vi "case_torture.vi"(7 "Main VI reference":refnum<vi>, 8 "error in (no error)":errorcluster, 10 "queue in":refnum<queue>, 11 "VISA resource name in":refnum<visa-resource-name>) -> (0 "error out":errorcluster, 3 "VISA Refnum out":refnum<visa-resource-name>)   [LabVIEW 2020]
uses:
  controls/message cluster.ctl
  <instrlib>/Marlin Instrument Driver/Public/controls/move parameters.ctl
  6b4587bc-0fd2-4684-895c-966bfeff11c4.vi
  3dbca1fd-0638-40ad-b8cf-a0dccebfc0b9.vi
  16951a91-4322-4001-be28-78344395b4b7.vi
  74ea327f-2ce8-422c-9958-5bfd1753f00f.vi
  50b149f9-9e82-4165-acdf-462a277af1c9.vi
  374137ba-4f25-4847-9236-12953adebbe7.vi
  f821f635-f9e4-4ceb-808f-b90ab8643010.vi
  <instrlib>/Marlin Instrument Driver/Marlin Instrument Driver.lvlib
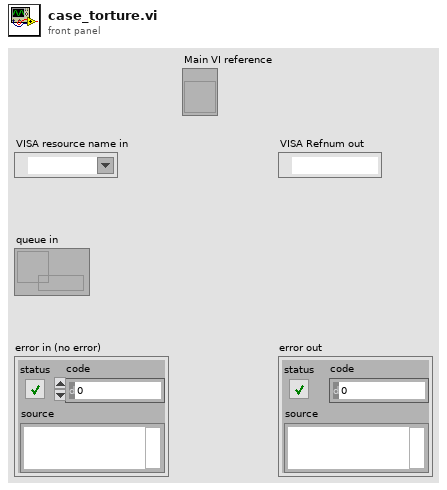
[diagram p1: front panel]
types:
  T1 = typedef "message cluster.ctl" = cluster{"message":string, "data":variant}
  T2 = typedef "Marlin Instrument Driver.lvlib/move parameters.ctl" = cluster{"E":dbl, "F":dbl, "X":dbl, "Y":dbl, "Z":dbl}
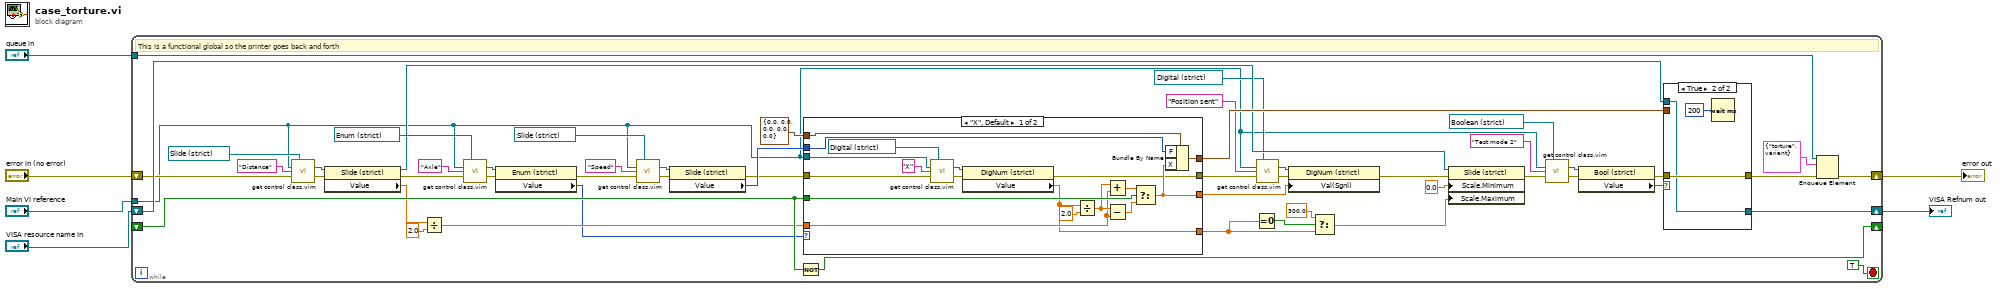
[diagram p0: block diagram]
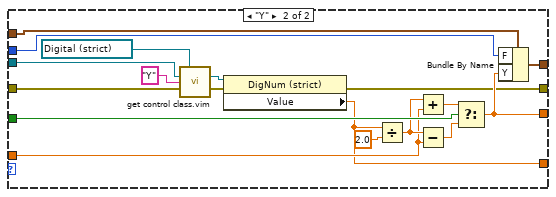
[diagram p2: hidden frame]
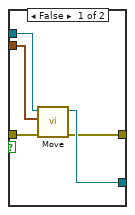
[diagram p3: hidden frame]
diagram:
  n1 = while {
    tunnel: "queue in" -> [w49]
    tunnel: "Main VI reference" -> [w7]
    shift-right: [w54] -> _
    shift-left: _ -> [w53]
    shift-right: [w45] -> w4
    shift-left: "VISA resource name in" -> [w44]
    shift-right: [w48] -> w5
    shift-left: "error in (no error)" -> [w24]
    stop <- TRUE stop-if-true
    # "This is a functional global so the printer goes back and forth"
    n2 = call "get control class.vim"("Control class"=refnum<vi> refnum ("Distance"), "Main VI reference"=w7, "Label"="Distance", "error in (no error)"=w24) -> ("Control out"=w27:refnum<vi>, "error out"=w26:errorcluster)  [unwired: 10 in]
    n3 = property class="Slide (strict)"(reference=w27, error in=w26) -> (reference out=w22:refnum<vi>, error out=w23:errorcluster, "Value"=w25:dbl)
    n4 = Divide(x=w25, y=2.0) -> (x/y=w52:dbl)
    n5 = call "get control class.vim"("Control class"=refnum<vi> refnum ("Axle"), "Main VI reference"=w7, "Label"="Axle", "error in (no error)"=w23) -> ("Control out"=w36:refnum<vi>, "error out"=w37:errorcluster)  [unwired: 10 in]
    n6 = property on="Property Node" class="Enum (strict)"(reference=w36, error in=w37) -> (error out=w16:errorcluster, "Value"=w50:enum16{"X", "Y", "Z"})  [unwired: 1 out]
    n7 = call "get control class.vim"("Control class"=refnum<vi> refnum ("Speed"), "Main VI reference"=w7, "Label"="Speed", "error in (no error)"=w16) -> ("Control out"=w19:refnum<vi>, "error out"=w20:errorcluster)  [unwired: 10 in]
    n8 = property on="Property Node" class="Slide (strict)"(reference=w19, error in=w20) -> (error out=w15:errorcluster, "Value"=w17:u32)  [unwired: 1 out]
    n9 = Not(x=w53) -> (.not. x?=w54:bool)
    n10 = case shown="\"X\", Default" w50 {
      tunnel: T2 {"E"=0.0, "F"=0.0, "X"=0.0, "Y"=0.0, "Z"=0.0} ("Distances") -> [w77 w94]
      tunnel: [w76 w95] -> w43
      tunnel: w17 -> [w75 w93]
      tunnel: w52 -> [w69 w87]
      tunnel: w53 -> [w71 w89]
      tunnel: [w68 w86] -> w59
      tunnel: [w67 w85] -> w10
      tunnel: w15 -> [w62 w80]
      tunnel: [w61 w79] -> w9
      tunnel: w7 -> [w60 w78]
      frame "X", Default {
        n11 = call "get control class.vim"("Control class"=refnum<vi> refnum ("X"), "Main VI reference"=w60, "Label"="X", "error in (no error)"=w62) -> ("Control out"=w64:refnum<vi>, "error out"=w63:errorcluster)  [unwired: 10 in]
        n12 = property on="Property Node" class="DigNum (strict)"(reference=w64, error in=w63) -> (error out=w61:errorcluster, "Value"=w68:dbl)  [unwired: 1 out]
        n13 = Divide(x=w68, y=2.0) -> (x/y=w70:dbl)
        n14 = Add(x=w70, y=w69) -> (x+y=w73:dbl)
        n15 = Subtract(x=w70, y=w69) -> (x-y=w72:dbl)
        n16 = Select(t=w73, s=w71, f=w72) -> (s? t:f=w67:dbl)
        n17 = Bundle By Name(cluster=w77, "F"=w75, "X"=w67) -> (w76:T2)
      }
      frame "Y" {
        n18 = call "get control class.vim"("Control class"=refnum<vi> refnum ("X"), "Main VI reference"=w78, "Label"="Y", "error in (no error)"=w80) -> ("Control out"=w82:refnum<vi>, "error out"=w81:errorcluster)  [unwired: 10 in]
        n19 = property on="Property Node" class="DigNum (strict)"(reference=w82, error in=w81) -> (error out=w79:errorcluster, "Value"=w86:dbl)  [unwired: 1 out]
        n20 = Divide(x=w86, y=2.0) -> (x/y=w88:dbl)
        n21 = Add(x=w88, y=w87) -> (x+y=w91:dbl)
        n22 = Subtract(x=w88, y=w87) -> (x-y=w90:dbl)
        n23 = Select(t=w91, s=w89, f=w90) -> (s? t:f=w85:dbl)
        n24 = Bundle By Name(cluster=w94, "F"=w93, "Y"=w85) -> (w95:T2)
      }
    }
    n25 = Equal To 0?(x=w59) -> (x = 0?=w56:bool)
    n26 = call "get control class.vim"("Control class"=refnum<vi> refnum ("X"), "Main VI reference"=w7, "Label"="Position sent", "error in (no error)"=w9) -> ("Control out"=w12:refnum<vi>, "error out"=w11:errorcluster)  [unwired: 10 in]
    n27 = property on="Property Node" class="DigNum (strict)"(reference=w12, error in=w11, "Val(Sgnl)"=w10) -> (error out=w8:errorcluster)  [unwired: 1 out]
    n28 = Select(t=300.0, s=w56, f=w59) -> (s? t:f=w57:dbl)
    n29 = property on="Property Node" class="Slide (strict)"(reference=w22, error in=w8, "Scale.Minimum"=0.0 ("Scale.Range:Minimum"), "Scale.Maximum"=w57) -> (error out=w31:errorcluster)  [unwired: 1 out]
    n30 = call "get control class.vim"("Control class"=refnum<vi> refnum ("Test mode 2"), "Main VI reference"=w7, "Label"="Test mode 2", "error in (no error)"=w31) -> ("Control out"=w33:refnum<vi>, "error out"=w32:errorcluster)  [unwired: 10 in]
    n31 = property class="Bool (strict)"(reference=w33, error in=w32) -> (error out=w29:errorcluster, "Value"=w30:bool)  [unwired: 1 out]
    n32 = case shown="True" w30 {
      tunnel: w43 -> [w100 _]
      tunnel: w29 -> [w99 w102]
      tunnel: w44 -> [w98 w101]
      tunnel: [w97 w101] -> w45
      tunnel: [w96 w102] -> w47
      frame False {
        n33 = call <instrlib>:"Move.vi"("error in (no error)"=w99, "Distances"=w100, "VISA resource name"=w98) -> ("error out"=w96:errorcluster, "VISA resource name out"=w97:refnum<visa-resource-name>)  [unwired: 7 in]
      }
      frame True {
        n34 = Wait (ms)(milliseconds to wait=u32 200) -> ()  [unwired: 1 out]
      }
    }
    n35 = Enqueue Element(queue=w49, element=T1 {"message"="torture", "data"=variant}, error in (no error)=w47) -> (error out=w48:errorcluster)  [unwired: 1 in, 2 out]
  }
  "error out" <- w5
  "VISA Refnum out" <- w4
